vi "Add Instr CFG.vi"(8 "error in (no error)":errorcluster, 10 "Instr Configuration":string, 11 "IConfiguration UI Actor in":refnum<class "IConfiguration UI Actor.lvclass">) -> (0 "error out":errorcluster, 3 "IConfiguration UI Actor out":refnum<class "IConfiguration UI Actor.lvclass">)   [LabVIEW 2024, in "IConfiguration UI Actor.lvlib" / "IConfiguration UI Actor.lvclass"]
uses:
  IConfiguration UI Actor.lvclass
  <vilib>/Utility/error.llb/Error Cluster From Error Code.vi
  <vilib>/ErrorRing/Error Ring.xnode
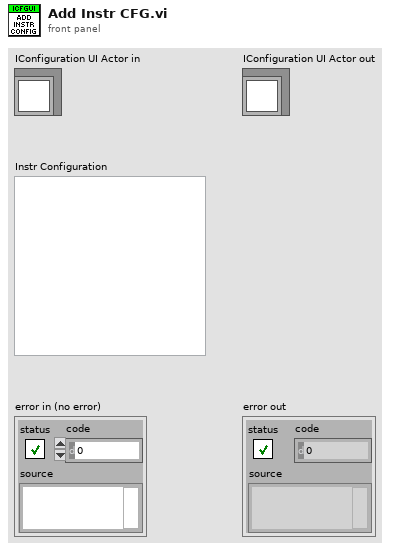
[diagram p1: front panel]
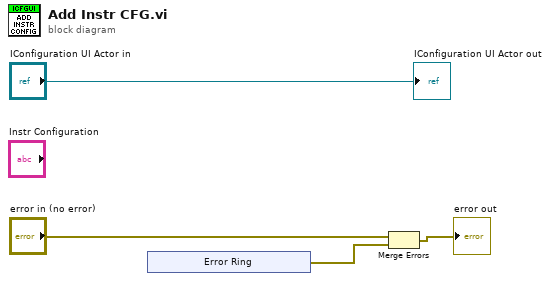
[diagram p0: block diagram]
diagram:
  n1 = xnode "Error Ring"() -> ("error out"=w1:errorcluster)
  n2 = Merge Errors("error in (no error)", w1) -> (→"error out":errorcluster)
  "IConfiguration UI Actor out" <- "IConfiguration UI Actor in"
